vi "To Path.vi"(10 "File in":refnum<class "File.lvclass">) -> (2 "Path out":path)   [LabVIEW 2020, in "Save for Previous Version.lvlib" / "File.lvclass"]
uses:
  File.lvclass
  File.lvclass/File.ctl
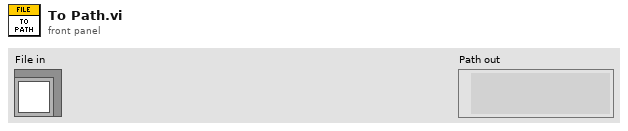
[diagram p1: front panel]
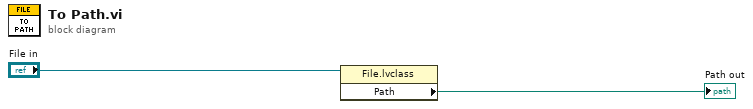
[diagram p0: block diagram]
diagram:
  n1 = property class="File.lvclass"(reference="File in") -> ("Path"=→"Path out":path)  [unwired: 1 in, 2 out]
